vi "Create.vi"(0 "Test Log Factory in":refnum<class "Test Log Factory.lvclass">, 5 "Test Log Types":T1, 7 "Test Name":string, 9 "Scan Name":string, 11 "error in (no error)":errorcluster) -> (4 "Test Log Factory out":refnum<class "Test Log Factory.lvclass">, 6 "Test Log":refnum<class "Test Log.lvclass">, 15 "error out":errorcluster)   [LabVIEW 2015, in "Test Log Factory.lvclass"]
uses:
  Test Log Factory.lvclass
  Test Log/Test Log.lvclass
  Typedefs/TestLogTypes.ctl
  Common_ConfigurationReader/ConfigurationReader.lvclass
  CSV Test Log/CSV Test Log.lvclass
  Typedefs/LogPath.ctl
  View/FAMT Views.lvlib
  Typedefs/FAMT Typedefs.lvlib
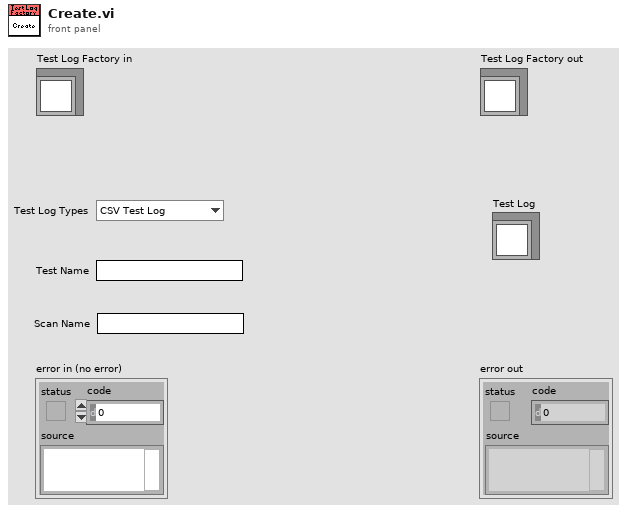
[diagram p1: front panel]
types:
  T1 = typedef "FAMT Typedefs.lvlib/TestLogTypes.ctl" = enum16{"CSV Test Log"}
  T2 = typedef "FAMT Typedefs.lvlib/LogPath.ctl" = path
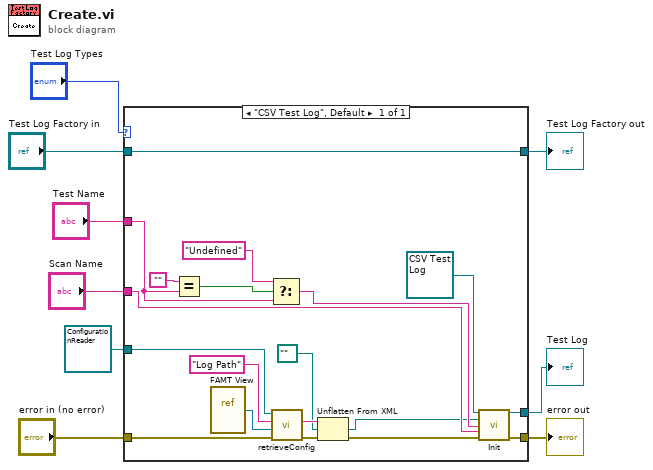
[diagram p0: block diagram]
diagram:
  n1 = case shown="\"CSV Test Log\", Default" "Test Log Types" {
    tunnel: "error in (no error)" -> [w23]
    tunnel: [w27] -> w3
    tunnel: [w18] -> w4
    tunnel: [w28] -> w2
    tunnel: "Test Log Factory in" -> [w28]
    tunnel: refnum<class "ConfigurationReader.lvclass"> refnum ("ConfigurationReader.lvclass") -> [w25]
    tunnel: "Test Name" -> [w14]
    tunnel: "Scan Name" -> [w11]
    frame "CSV Test Log", Default {
      n2 = Equal?(x="", y=w14) -> (x = y?=w15:bool)
      n3 = vi-ref "FAMT View.vi"() -> (w17:refnum<vi>)
      n4 = Select(t="Undefined", s=w15, f=w14) -> (s? t:f=w13:string)
      n5 = call "retrieveConfig.vi"("error in (no error)"=w23, "callingVIRef"=w17, "configName"="Log Path", "ConfigurationReader in"=w25) -> ("error out"=w21:errorcluster, "xmlData"=w22:string)  [unwired: 5 in, 1 out]
      n6 = Unflatten From XML(xml string=w22, type=T2 path "" ("Log Path"), error in (no error)=w21) -> (value=w10:T2, error out=w19:errorcluster)
      n7 = call "Init.vi"("CSV Test Log in"=refnum<class "CSV Test Log.lvclass"> refnum ("CSVTestLog.lvclass"), "Log Path"=w10, "Test Name"=w13, "Scan Name"=w11, "error in (no error)"=w19) -> ("CSV Test Log out"=w27:refnum<class "CSV Test Log.lvclass">, "error out"=w18:errorcluster)  [unwired: 9 in]
    }
  }
  "error out" <- w4
  "Test Log Factory out" <- w2
  "Test Log" <- w3
